vi "Main_23a.vi"() -> ()   [LabVIEW 2023]
uses:
  RB ENUM_Spot ID.ctl
  Cluster _Point Location.ctl
  ENUM_Location Direction.ctl
panel:
  in  "Description":string="--- Day 23: Unstable Diffusion ---\nYou enter a large crater of gray dirt where the grove is supposed to be. All around you, plants you imagine were expected to be full of fruit are instead withered and broken. A large group of Elves has formed in the middle of the grove.\n\n\"...but this volcano has been dormant for months. Without ash, the fruit can't grow!\"\n\nYou look up to see a massive, snow-capped mountain towering above you.\n\n\"It's not like there are other active volcanoes here; we've looked everywhere.\"\n\n\"But our scanners show active magma flows; clearly it's going somewhere.\"\n\nThey finally notice you at the edge of the grove, your pack almost overflowing from the random star fruit you've been collecting. Behind you, elephants and monkeys explore the grove, looking concerned. Then, the Elves recognize the ash cloud slowly spreading above your recent detour.\n\n\"Why do you--\" \"How is--\" \"Did you just--\"\n\nBefore any of them can form a complete question, another Elf speaks up: \"Okay, new plan. We have almost enough fruit already, and ash from the plume should spread here eventually. If we quickly plant new seedlings now, we can still make it to the extraction point. Spread out!\"\n\nThe Elves each reach into their pack and pull out a tiny plant. The plants rely on important nutrients from the ash, so they can't be planted too close together.\n\nThere isn't enough time to let the Elves figure out where to plant the seedlings themselves; you quickly scan the grove (your puzzle input) and note their positions.\n\nFor example:\n\n....#..\n..###.#\n#...#.#\n.#...##\n#.###..\n##.#.##\n.#..#..\nThe scan shows Elves # and empty ground .; outside your scan, more empty ground extends a long way in every direction. The scan is oriented so that north is up; orthogonal directions are written N (north), S (south), W (west), and E (east), while diagonal directions are written NE, NW, SE, SW.\n\nThe Elves follow a time-consuming process to figure out where they should each go; you can speed up this process considerably. The process consists of some number of rounds during which Elves alternate between considering where to move and actually moving.\n\nDuring the first half of each round, each Elf considers the eight positions adjacent to themself. If no other Elves are in one of those eight positions, the Elf does not do anything during this round. Otherwise, the Elf looks in each of four directions in the following order and proposes moving one step in the first valid direction:\n\nIf there is no Elf in the N, NE, or NW adjacent positions, the Elf proposes moving north one step.\nIf there is no Elf in the S, SE, or SW adjacent positions, the Elf proposes moving south one step.\nIf there is no Elf in the W, NW, or SW adjacent positions, the Elf proposes moving west one step.\nIf there is no Elf in the E, NE, or SE adjacent positions, the Elf proposes moving east one step.\nAfter each Elf has had a chance to propose a move, the second half of the round can begin. Simultaneously, each Elf moves to their proposed destination tile if they were the only Elf to propose moving to that position. If two or more Elves propose moving to the same position, none of those Elves move.\n\nFinally, at the end of the round, the first direction the Elves considered is moved to the end of the list of directions. For example, during the second round, the Elves would try proposing a move to the south first, then west, then east, then north. On the third round, the Elves would first consider west, then east, then north, then south.\n\nAs a smaller example, consider just these five Elves:\n\n.....\n..##.\n..#..\n.....\n..##.\n.....\nThe northernmost two Elves and southernmost two Elves all propose moving north, while the middle Elf cannot move north and proposes moving south. The middle Elf proposes the same destination as the southwest Elf, so neither of them move, but the other three do:\n\n..##.\n.....\n..#..\n...#.\n..#..\n.....\nNext, the northernmost two Elves and the southernmost Elf all propose moving south. Of the remaining middle two Elves, the west one cannot move south and proposes moving west, while the east one cannot move south or west and proposes moving east. All five Elves succeed in moving to their proposed positions:\n\n.....\n..##.\n.#...\n....#\n.....\n..#..\nFinally, the southernmost two Elves choose not to move at all. Of the remaining three Elves, the west one proposes moving west, the east one proposes moving east, and the middle one proposes moving north; all three succeed in moving:\n\n..#..\n....#\n#....\n....#\n.....\n..#..\nAt this point, no Elves need to move, and so the process ends.\n\nThe larger example above proceeds as follows:\n\n== Initial State ==\n..............\n..............\n.......#......\n.....###.#....\n...#...#.#....\n....#...##....\n...#.###......\n...##.#.##....\n....#..#......\n..............\n..............\n..............\n\n== End of Round 1 ==\n..............\n.......#......\n.....#...#....\n...#..#.#.....\n.......#..#...\n....#.#.##....\n..#..#.#......\n..#.#.#.##....\n..............\n....#..#......\n..............\n..............\n\n== End of Round 2 ==\n..............\n.......#......\n....#.....#...\n...#..#.#.....\n.......#...#..\n...#..#.#.....\n.#...#.#.#....\n..............\n..#.#.#.##....\n....#..#......\n..............\n..............\n\n== End of Round 3 ==\n..............\n.......#......\n.....#....#...\n..#..#...#....\n.......#...#..\n...#..#.#.....\n.#..#.....#...\n.......##.....\n..##.#....#...\n...#..........\n.......#......\n..............\n\n== End of Round 4 ==\n..............\n.......#......\n......#....#..\n..#...##......\n...#.....#.#..\n.........#....\n.#...###..#...\n..#......#....\n....##....#...\n....#.........\n.......#......\n..............\n\n== End of Round 5 ==\n.......#......\n..............\n..#..#.....#..\n.........#....\n......##...#..\n.#.#.####.....\n...........#..\n....##..#.....\n..#...........\n..........#...\n....#..#......\n..............\nAfter a few more rounds...\n\n== End of Round 10 ==\n.......#......\n...........#..\n..#.#..#......\n......#.......\n...#.....#..#.\n.#......##....\n.....##.......\n..#........#..\n....#.#..#....\n..............\n....#..#..#...\n..............\nTo make sure they're on the right track, the Elves like to check after round 10 that they're making good progress toward covering enough ground. To do this, count the number of empty ground tiles contained by the smallest rectangle that contains every Elf. (The edges of the rectangle should be aligned to the N/S/E/W directions; the Elves do not have the patience to calculate arbitrary rectangles.) In the above example, that rectangle is:\n\n......#.....\n..........#.\n.#.#..#.....\n.....#......\n..#.....#..#\n#......##...\n....##......\n.#........#.\n...#.#..#...\n............\n...#..#..#..\nIn this region, the number of empty ground tiles is 110.\n\nSimulate the Elves' process and find the smallest rectangle that contains the Elves after 10 rounds. How many empty ground tiles does that rectangle contain?"
  out "Elf Locations":T1[](array[typedef])
  out "Grove":T2[][](array[typedef])
  in  "Example 2":string="....#..\n..###.#\n#...#.#\n.#...##\n#.###..\n##.#.##\n.#..#.."
  out "Answer":u32
  in  "Puzzle":string="###.###...#.##.###.##.###.....#...##.#####..####..#####.#...###..##...#..\n####.#..#..#..#.###..###....###.....#.#.##.###.#..#..#..##########..#..#.\n.##..##..#.##.#.....##.##..#..###..#..#.####...##...#...##.#...#.#....###\n###.#..#.#..#...###.#...#..##.#.#####..#...###.##..#....##..#......##..#.\n.#..##.#.##..##.####.###.###...###.##.#.###.#...####.#######..#..##.#####\n#...#.#.#####...#.#...###...#.#....#..#..##....##...####.####..#.########\n#..######..#.#..#..##......#..##.######....#.....###..######...#.#.###...\n.###.####.#.#.###.#.....#...##..#...#.#.#.#.####.#..#..#.##..##..##.#.#.#\n#.#..#.####....#.##.#........#....#.###.##...##......#...#..####.#.#.#.#.\n###.#..##...#.#.#.##.##....#.#..#....######...#...##.#.####..#...##.#..#.\n#...###..#.##..#.#.#...##..#.#.....#..#..#.#...#...#####..#.##..#.##.####\n..#.#.#....#..#..###.#...#.#..#.#.#..#....###...###......#.#.#...#.######\n###.###.###.#.#...####.###..#.#..#....#..#.###........#....##.#.....###..\n#..#..#..#.###...#.##.##...#.##.#.#.#.#.###.#.##..#..##.#.####.#####..#.#\n.###.##..###.....#.#..#.#..###..#.#..#.#...##.#.....##...####..#.#.##.##.\n#.###.##.##.####.###.#.#.#..##..####...#####...###..#.##..##.##.###.##.#.\n#.####.####.#..#######..###...#.....##.###.#.##.#.##.###.....#..#..#...#.\n..###.##..######..#....#.#.#....#..#..#.#.####..#....####.##.##.#.#######\n#..##.#..####..######.####.#..#.#..##...###.###.####.#.....##.#####..##..\n.##..#...##..###..####.##.########.#.#....#.##..##.#.........#...########\n##..###..#....#.###.##.#.#...###.###.##.#...##..#..#.###.##.#.##...##...#\n.#...##.###..#.########.#....#.##......#...#.##..##..#.###..##.......##.#\n#.#.....#####..#.#..#####.##..###..#.##.##..#..#.......##.#.##.##..######\n#.##.#.##.###.#..########..##.#.#.#######....###.....###.#...#.##....##..\n.#..#...#.###.#.#..#..#.....#..##...##.#.#####.#...##....##...#.......###\n...#...#####..########.####.######.####..#.#.#.##.#.###...#.##.###..#...#\n.#.#.####.###...##.####.......#..#..#...#......######.##.#...#.#...######\n#.....##.###.###.###.##.....#..#######....#..#.#...##.#..#..###.#..#.#..#\n.#...##.#...###.###.##...##..#.#.####.#.##..#.##.#.#.####....#.#.#.#.####\n.#######.#.....##.####...##..##.###...##.##.#..#..#...#..#####.#.###..##.\n....##.......#...#.###.#####..#.#.##.#.#.##..#.##.#####.##.##.#..##.###..\n###.#.##...#.#.####.####..##...##..##.#.#.#.#...###.##.###.##..#...#...#.\n.#.##.#....##..#.##...##.###..###..#.#..#.#########.....#.##...##....#.#.\n..##.#..###..#.......#....#.#.#.###.###.#.#..#.#.#..#...#.###.##..####...\n.##.##.#.###...#.##....#.##..###..#..###..###.#...##.....#.###.#.####..#.\n....#..##..#.......####.##.#.##.###.#.#..######.###.##.#.#.###..####..#..\n####..#.###.##..##.##..#.###....####.###.#.#####.#.##.#.#...##.....##...#\n.#....#.##...#....#####....#.#######.#.###...###.#.##.#..#.##...#.#....#.\n#.###..####......###.##....#.#.####...#.#.#...###.#.........#.#.##......#\n#..#....#.#.##..##..#..#.###.###.#.###.#####..#..##.###...##.##..#.#....#\n#...##.#...##.#.##...##.#..#.#.##.##....#....#..##..###.#....####.######.\n....#.#...##.......#####...######..###...###.##.#.##.#.##..#.##.##....#..\n..####.###..#....##.##.############.#.##...####.###.#....#....##.#.######\n#...#.#####.#.##.#.##.##...###.....#..###.#.###.###........#....#...#....\n#...#....#...####..#.#..###....#..#######.#....##..##..#..#..##..#...####\n#.#.##.##.##.#.##.####..####.....##.....#.#.#.##..###.#.##.#...##.#..##..\n..#..##.#..###.....##.##...#.##..#.##...###.#.###.#..###.....#..##..#..##\n##.#.#.#.###...#....##.....######..#####.##..#..#..#.##.#.####..##.##.##.\n.##.##...#.##.#...##...####.#..#...#.#..#.###.##.##....#.##.#..#..#.#.###\n.###.#...###.##.#.#..###.##..###.#####.#..#####..###....###.##.#.#.#..###\n..###...#####...#...##..#.#.#...#.##....#..##.#..#.#.#...####..#.#.##..#.\n#.#.##.##.#.##...##.#.##.##.#.##.###..###..#.##..#.#..####.##.#.....##..#\n..#..###..#.#####..###.##......####.###..#.##.#.##..###..#.###..#####.#..\n.###.#...#.#.#.#####..###..###.#..##.###..##...###.#.#..#....##.#.#.##.#.\n#.##....####.##.##...###.##...######....#..##.#.#..#####...#...#.###.##..\n..#....##...#.#####....#......#.....#.#.#...#...#...##.#.#...##..#.#...##\n.#.#..##..######..##..#.#..#.........#.#..#....#.#......#.##..###.##.#..#\n####..#.#.#..#..##..#.#.####.###......#..#.....#..#.####..#.#####.#..#.##\n.##.#..##..###....#..#...#.#####....##..#......###...##.#...##....####..#\n..####.#..###.###.###...##..#.#......#####.#.#.#..##......###.#.#.###.##.\n#####....###.##..#.##..###########..#.#.#.#...##..#####.#.#..#..####..#.#\n##..#.##.#.##.....#.###.#.#.......##...#...#.#.##....#..#......#####..##.\n###.#...##.##..####.#...####..#.###.....#.###...#.#.##..#####......#.#.##\n#.##.#############.##....#.###.####.##.#.######.#.#....#..######..##.####\n.#.###.####.##...#..##....##..##.#..#.#...#####...####....#..#...###.#.#.\n.###..#..##...##..####...###.#..##########.###.##.#..###.#..###...##.#.##\n.##.##.#..#.####..#####......##.#..#....#.##..#.####.#.###########.#.#.#.\n..#.####.#...##.#.#....##.#...##..##...#.#.#.##..##..##.####..##.#####.#.\n.....#.##.####..##.#.##....#.##..##..##...#.#...##..#.#..####.###..#.#..#\n..#.....#####.##..###.#.###.....#.#.######.#.....###.....#..#.#...#..#.##\n#.#..#.#..##.#.#.....##.#.##..###.###.##..#..###..######..#.####.....##.#\n..####.......###.#..###.#.#.######.####.##...#.##...######..#####...#...#\n#.#.####.####..########.#.....##......#.##.##.#.#....##.####.##..#...####"
  in  "Example":string=".....\n..##.\n..#..\n.....\n..##.\n....."
  # "3990"
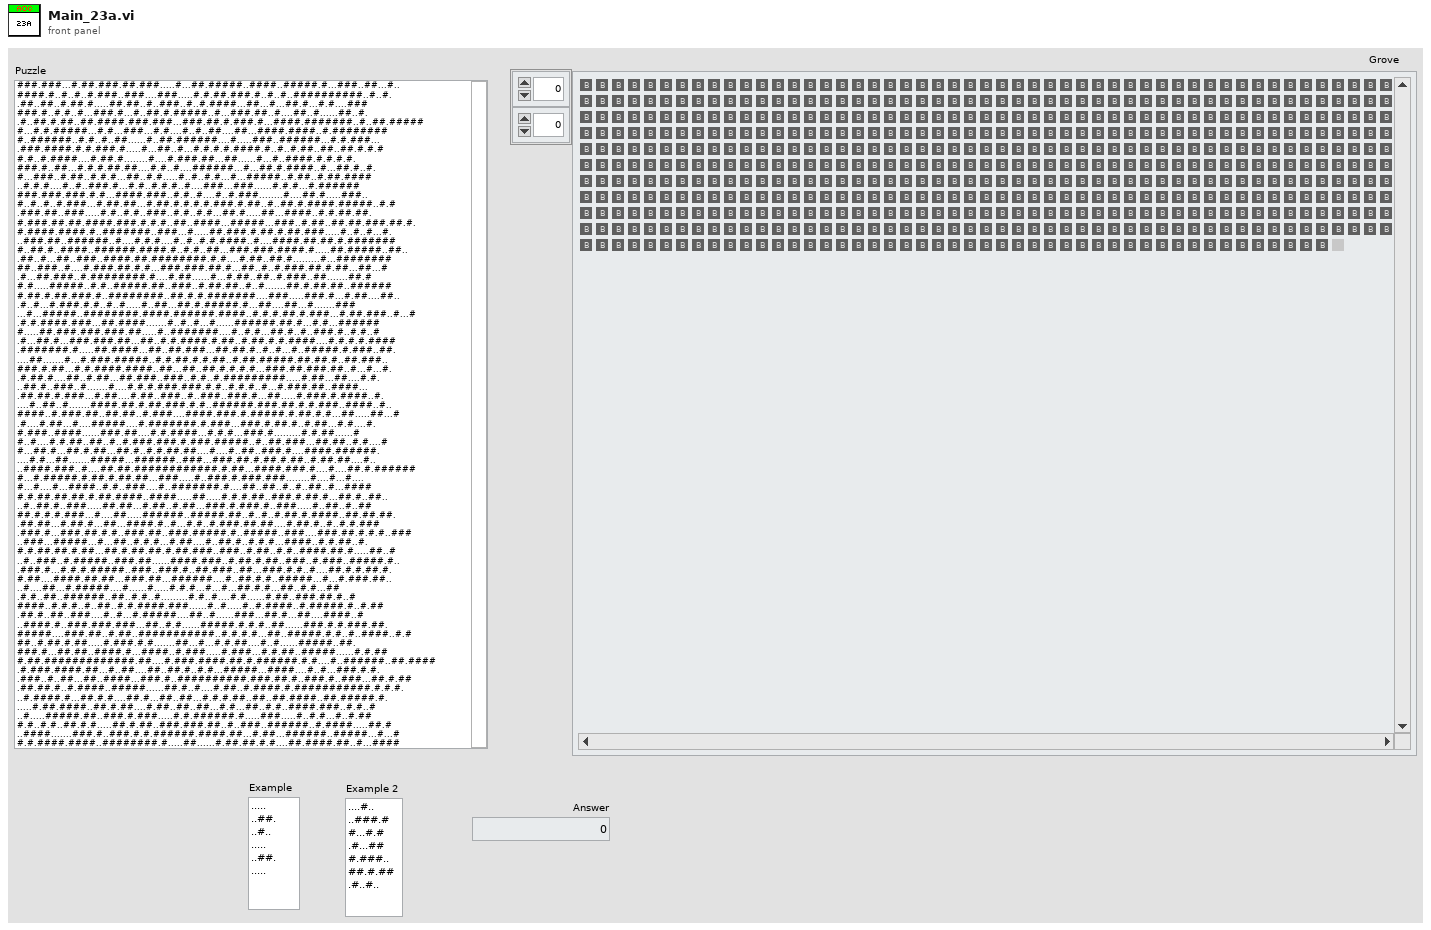
[diagram p1: front panel]
types:
  T1 = typedef "Cluster _Point Location.ctl" = cluster{"X col":i32, "Y row":i32}
  T2 = typedef "RB ENUM_Spot ID.ctl" = enum32{"Blank", "ELF", "Proposed"}
  T3 = typedef "ENUM_Location Direction.ctl" = enum16{"North", "North-East", "East", "South-East", "South", "South-West", "West", "North-West", "Center"}
  T4 = typedef "MAP_Poroposed Moves.ctl" = map{T1, cluster{"Elf":i32, "move":bool}}
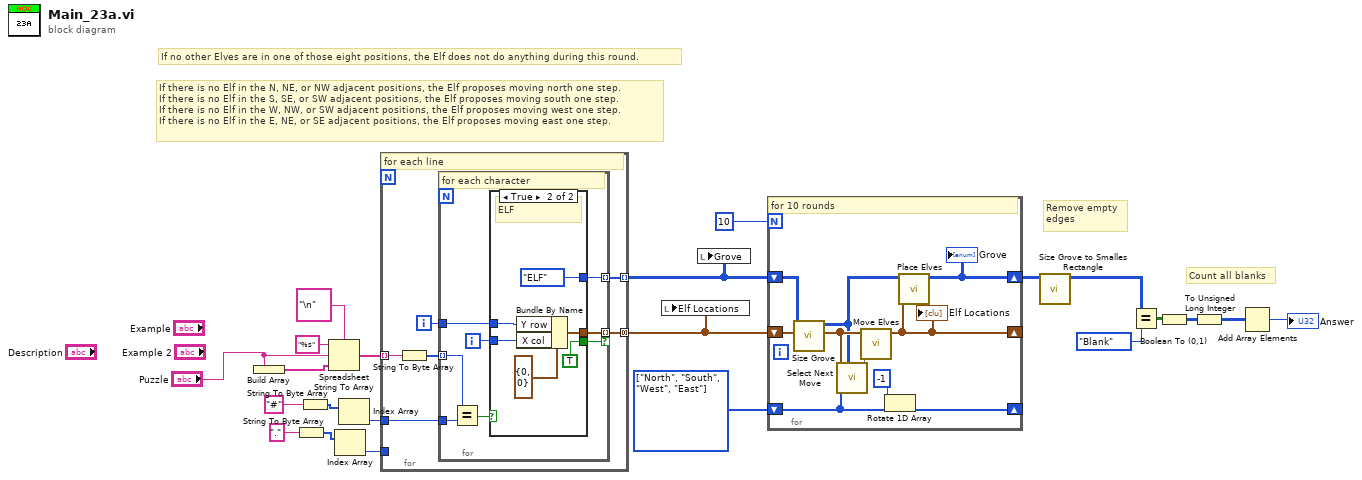
[diagram p0: block diagram]
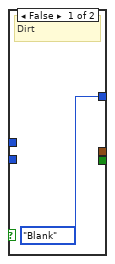
[diagram p2: hidden frame]
diagram:
  w11 = T3[] [enum."North", enum."South", enum."West", enum."East"] items=["North", "North-East", "East", "South-East", "South", "South-West", "West", "North-West", "Center"] ("Array")
  # "Count all blanks"
  # "Remove empty\nedges"
  # "If there is no Elf in the N, NE, or NW adjacent positions, the Elf proposes moving north one step.\nIf there is no Elf in the S, SE, or SW adjacent positions, the Elf proposes moving south one step.\nIf there is no Elf in the W, NW, or SW adjacent positions, the Elf proposes moving west one step.\nIf there is no Elf in the E, NE, or SE adjacent positions, the Elf proposes moving east one step."
  # "If no other Elves are in one of those eight positions, the Elf does not do anything during this round."
  n1 = Build Array("Puzzle") -> (w22:string[])
  n2 = String To Byte Array(string="." ("format string")) -> (unsigned byte array=w15:u8[])
  n3 = String To Byte Array(string="#" ("format string")) -> (unsigned byte array=w16:u8[])
  n4 = Spreadsheet String To Array(delimiter (Tab)="\n", format string="%s", spreadsheet string="Puzzle", array type (2D Dbl)=w22) -> (array=w19:string[])
  n5 = Index Array(array=w15) -> (element=w14:u8)  [unwired: 1 in]
  n6 = Index Array(array=w16) -> (element=w13:u8)  [unwired: 1 in]
  n7 = for {
    tunnel: w19 -> [w28] mode=indexing
    tunnel: w14 -> [_]
    tunnel: w13 -> [w26]
    tunnel: [w25] -> w10 mode=indexing
    tunnel: [w23] -> w9 mode=concatenating
    i -> [w24]
    # "for each line"
    n8 = String To Byte Array(string=w28) -> (unsigned byte array=w27:u8[])
    n9 = for {
      tunnel: w27 -> [w35] mode=indexing
      tunnel: w26 -> [w36]
      tunnel: [w33] -> w25 mode=indexing
      tunnel: w24 -> [w31]
      tunnel: [w30] -> w23 mode=indexing if=w29
      i -> [w32]
      # "for each character"
      n10 = Equal?(x=w35, y=w36) -> (x = y?=w34:bool)
      n11 = case shown="True" w34 {
        tunnel: [RB_ENUM_Spot_ID."Blank" ("Spot") RB_ENUM_Spot_ID."ELF" ("Spot")] -> w33
        tunnel: w32 -> [_ w41]
        tunnel: w31 -> [_ w40]
        tunnel: [_ w39] -> w30
        tunnel: [_ TRUE] -> w29
        frame False {
          # "Dirt"
        }
        frame True {
          # "ELF"
          n12 = Bundle By Name(cluster=T1 {"X col"=0, "Y row"=0} ("Point"), "Y row"=w40, "X col"=w41) -> (w39:T1)
        }
      }
    }
  }
  n13 = local write "Elf Locations"(w9) -> ()
  n14 = local write "Grove"(w10) -> ()
  n15 = for {
    N: 10 -> [_]
    shift-right: [w48] -> w8
    shift-left: w10 -> [w50]
    shift-right: [w47] -> _
    shift-left: w9 -> [w46]
    shift-right: [w53] -> _
    shift-left: w11 -> [w51]
    # "for 10 rounds"
    n16 = call "Size Grove.vi"("Elf Locations"=w46, "Original Grove"=w50) -> ("Elf Locations 2"=w45:T1[], "Spaced Grove"=w44:T2[][])  [unwired: 8 in]
    n17 = call "Select Next Move.vi"("Grove"=w44, "Proposed Direction List"=w51, "Elf"=w45) -> ("propose Moves"=w49:T4)  [unwired: 7 in, 1 out]
    n18 = call "Move Elves.vi"("propose Moves"=w49, "Elf Positions"=w45) -> ("New Elf Positions"=w47:T1[])  [unwired: 9 in]
    "Elf Locations" <- w47
    n19 = Rotate 1D Array(1:w51, 2:-1 ("n")) -> (0:w53:T3[])
    n20 = call "Place Elves.vi"("Elf Locations"=w47, "Spaced Grove in"=w44) -> ("Spaced Grove out"=w48:T2[][])  [unwired: 9 in]
    "Grove" <- w48
  }
  n21 = call "Size Grove to Smalles Rectangle.vi"("Grove"=w8) -> ("Sized Grove"=w7:T2[][])  [unwired: 10 in]
  n22 = Equal?(x=w7, y=RB_ENUM_Spot_ID."Blank" ("Spot")) -> (x = y?=w5:bool[][])
  n23 = Boolean To (0,1)(Boolean=w5) -> (0, 1=w4:i16[][])
  n24 = To Unsigned Long Integer(number=w4) -> (unsigned 32bit integer=w2:u32[][])
  n25 = Add Array Elements(numeric array=w2) -> (sum=→"Answer":u32)
